vi "Drive Controller.vi"(8 "error in":errorcluster) -> ()   [LabVIEW 2019]
doc: "This VI executes continuously carrying out the current operation and responding to updates or new operation requests. It will often contain the timing or control code that is difficult to place directly in TeleOp. This VI generally opens all sensors and motors and isolates the rest of the robot code from knowing implementation details of how the operations are carried out."
uses:
  Drive Setpoints.ctl
  Drive Operations.ctl
  <vilib>/Rock Robotics/WPI/Solenoid/WPI_SolenoidChannel.ctl
  <vilib>/Rock Robotics/WPI/SafetyOutput/WPI_SafetyOutputConfigMenu.ctl
  <vilib>/Rock Robotics/WPI/ThirdParty/Phoenix-LabVIEW/Motor Controller/Controls/CTRE_Phoenix_MotorControl_ControlMode.ctl
  <vilib>/Rock Robotics/WPI/ThirdParty/Phoenix-LabVIEW/Motor Controller/Controls/CTRE_Phoenix_MotorControl_NeutralMode.ctl
  <vilib>/Rock Robotics/WPI/ThirdParty/Phoenix-LabVIEW/Motor Controller/Controls/CTRE_Phoenix_MotorControl_FeedbackDevice.ctl
  <vilib>/Rock Robotics/WPI/ThirdParty/Phoenix-LabVIEW/Motor Controller/Controls/CTRE_Phoenix_MotorControl_StatusFrameEnhanced.ctl
  <vilib>/Rock Robotics/WPI/Solenoid/WPI_SolenoidValue.ctl
  <vilib>/Rock Robotics/WPI/Solenoid/WPI_SolenoidOpenSingle.vi
  <vilib>/Rock Robotics/WPI/Solenoid/WPI_SolenoidSetEnum.vi
  <vilib>/Rock Robotics/WPI/Utilities/WPI_GetSetVariantRefNum.vi
  <vilib>/Rock Robotics/WPI/RobotDrive/WPI_RobotDriveMecanumDrive_Cartesian.vi
  <vilib>/Rock Robotics/WPI/ThirdParty/Phoenix-LabVIEW/Motor Controller/Get/CTRE_Phoenix_MotorController_GetQuadratureData.vi
panel:
  in  "output range":cluster{"output high":dbl, "output low":dbl}={"output high"=0.5, "output low"=-0.5}
  in  "PID gains":T1={"proportional gain (Kc)"=0.035, "integral time (Ti, min)"=0.0, "derivative time (Td, min)"=0.0018}
  out "Current\nCmd":string
  # ".578"
  # "Tip: It may be helpful to observe inputs and sensor values.\nYou may also want to display tuning or debugging controls."
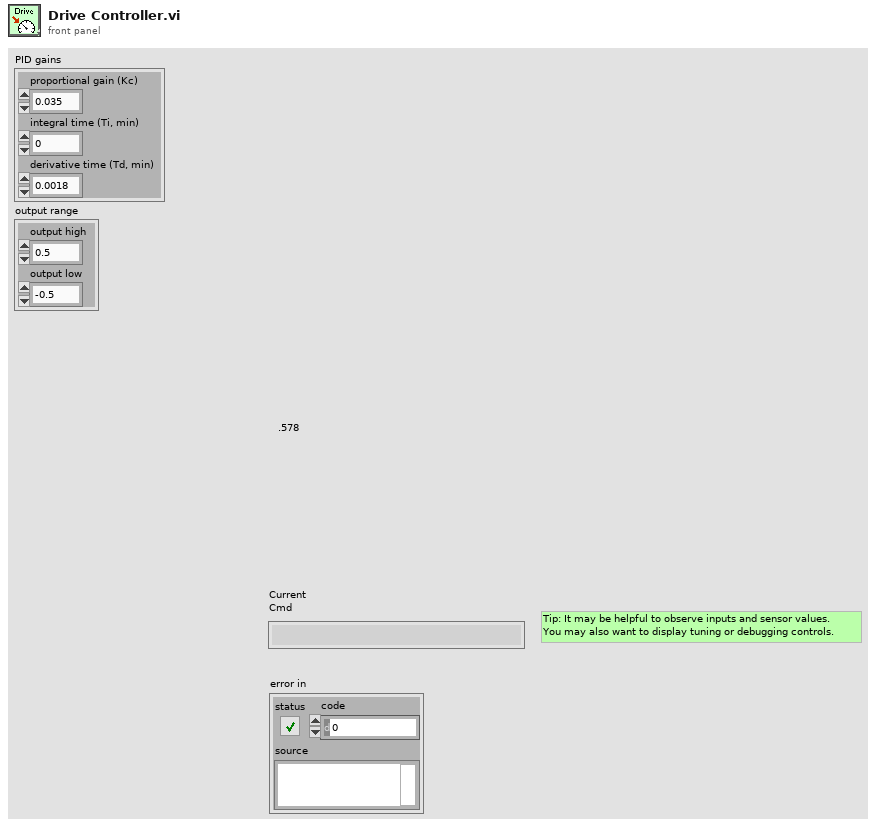
[diagram p1: front panel]
types:
  T1 = cluster{"proportional gain (Kc)":dbl, "integral time (Ti, min)":dbl, "derivative time (Td, min)":dbl}
  T2 = typedef "CTRE_Phoenix_MotorControl_StatusFrameEnhanced.ctl" = u16
  T3 = typedef "WPI_SolenoidChannel.ctl" = enum8{"Solenoid 0", "Solenoid 1", "Solenoid 2", "Solenoid 3", "Solenoid 4", "Solenoid 5", "Solenoid 6", "Solenoid 7", "Invalid"}
  T4 = typedef "CTRE_Phoenix_MotorControl_FeedbackDevice.ctl" = i8
  T5 = typedef "CTRE_Phoenix_MotorControl_NeutralMode.ctl" = enum8{"EEPROMSetting", "Override to Coast", "Override to Brake"}
  T6 = typedef "CTRE_Phoenix_MotorControl_ControlMode.ctl" = u16
  T7 = typedef "WPI_SafetyOutputConfigMenu.ctl" = enum16{"Enable", "Disable"}
  T8 = typedef "Drive Setpoints.ctl" = cluster{"Operation":T9, "X Setpoint":dbl, "Y Setpoint":dbl, "Duration":dbl, "Z Setpoint":dbl, "Tracks":bool, "Gyro":dbl, "POV":i16, "Distance(feet)":dbl, "AutoTrack Toggle":bool, "Collsision Detection":bool, "Reset Encoder":bool, "MP File Name":string}
  T9 = typedef "Drive Operations.ctl" = enum16{"Reserve", "Read Current", "Reset Motors VBus", "Motion Profile run", "Immediate Robot Centric", "Drive for Time Robot Centric", "Immediate Field Centric", "Drive For Time Field Centric", "Button Adjust", "Set Motors Motion Profile", "Reset Encoders", "Motion Profile Enable", "Drive for Distance"}
  T10 = typedef "WPI_MotorControlDeviceRef.ctl" = cluster{"DeviceStatus":errorcluster, "Type":T11, "PWM":cluster{"PWM Channel":T12, "DeadBand":T13}, "CAN":cluster{"Device Number":u8, "SetOutput VI Ref":variant, "GetOutput VI Ref":variant, "Enable VI Ref":variant, "Disable VI Ref":variant, "Data":variant}, "Invert":bool, "DIO PWM":cluster{"PWM \"Enable\" Channel":T12, "DIOChannel":T14, "PWM Rate":dbl}}
  T11 = typedef "WPI_MotorControlType.ctl" = enum16{"PWM", "CAN", "DIO PWM"}
  T12 = typedef "FPGA_DIOPWMChannel.ctl" = enum8{"PWM 0", "PWM 1", "PWM 2", "PWM 3", "PWM 4", "PWM 5", "PWM 6", "PWM 7", "PWM 8", "PWM 9", "PWM MXP 0", "PWM MXP 1", "PWM MXP 2", "PWM MXP 3", "PWM MXP 4", "PWM MXP 5", "PWM MXP 6", "PWM MXP 7", "PWM MXP 8", "PWM MXP 9", "Invalid"}
  T13 = typedef "WPI_PWMDeadband.ctl" = cluster{"Name":string, "maxPositivePwm":i32, "minPositivePwm":i32, "centerPwm":i32, "maxNegativePwm":i32, "minNegativePwm":i32, "angularRange":u16}
  T14 = typedef "FPGA_DIOChannel.ctl" = enum8{"DIO 0", "DIO 1", "DIO 2", "DIO 3", "DIO 4", "DIO 5", "DIO 6", "DIO 7", "DIO 8", "DIO 9", "DIO MXP 0", "DIO MXP 1", "DIO MXP 2", "DIO MXP 3", "DIO MXP 4", "DIO MXP 5", "DIO MXP 6", "DIO MXP 7", "DIO MXP 8", "DIO MXP 9", "DIO MXP 10", "DIO MXP 11", "DIO MXP 12", "DIO MXP 13", "DIO MXP 14", "DIO MXP 15", "SPI Port CS1", "SPI Port CS2", "SPI Port CS3", "SPI Port MISO", "SPI Port MOSI", "Invalid"}
  T15 = typedef "WPI_RobotDriveDevRef.ctl" = cluster{"DevStatus":errorcluster, "Motors[]":T10[], "Square Inputs":bool, "Max Output":dbl}
  T16 = typedef "WPI_SolenoidDevRef.ctl" = cluster{"DevStatus":errorcluster, "Pneumatics Control Module":u8, "Forward Solenoid Channel":T3, "Reverse Solenoid Channel":T3}
  T17 = typedef "Command Status Info.ctl" = cluster{"Name":string, "Status":T18, "notifier out":T19}
  T18 = typedef "Completion Status.ctl" = enum16{"Successful", "Aborted", "Incomplete"}
  T19 = typedef "Completion Notifier.ctl" = refnum<notifier>
  T20 = cluster{"SubSystem Data":T8, cluster{"Start Time (ms)":u32, "Iterations":i32}, cluster{"Command Info":T17, "Description":string, "SubSystem Data":T8, "notifier out":refnum<notifier>, "Subsystem Name":string}}
  T21 = typedef "WPI_SolenoidValue.ctl" = enum16{"Off", "On", "Forward", "Reverse"}
  T22 = cluster{"SubSystem Data":T8, cluster{"Start Time (ms)":u32, "Iterations":i32}, "Default Command Arguments":cluster{"Command Info":T17, "Description":string, "SubSystem Data":T8, "notifier out":refnum<notifier>, "Subsystem Name":string}}
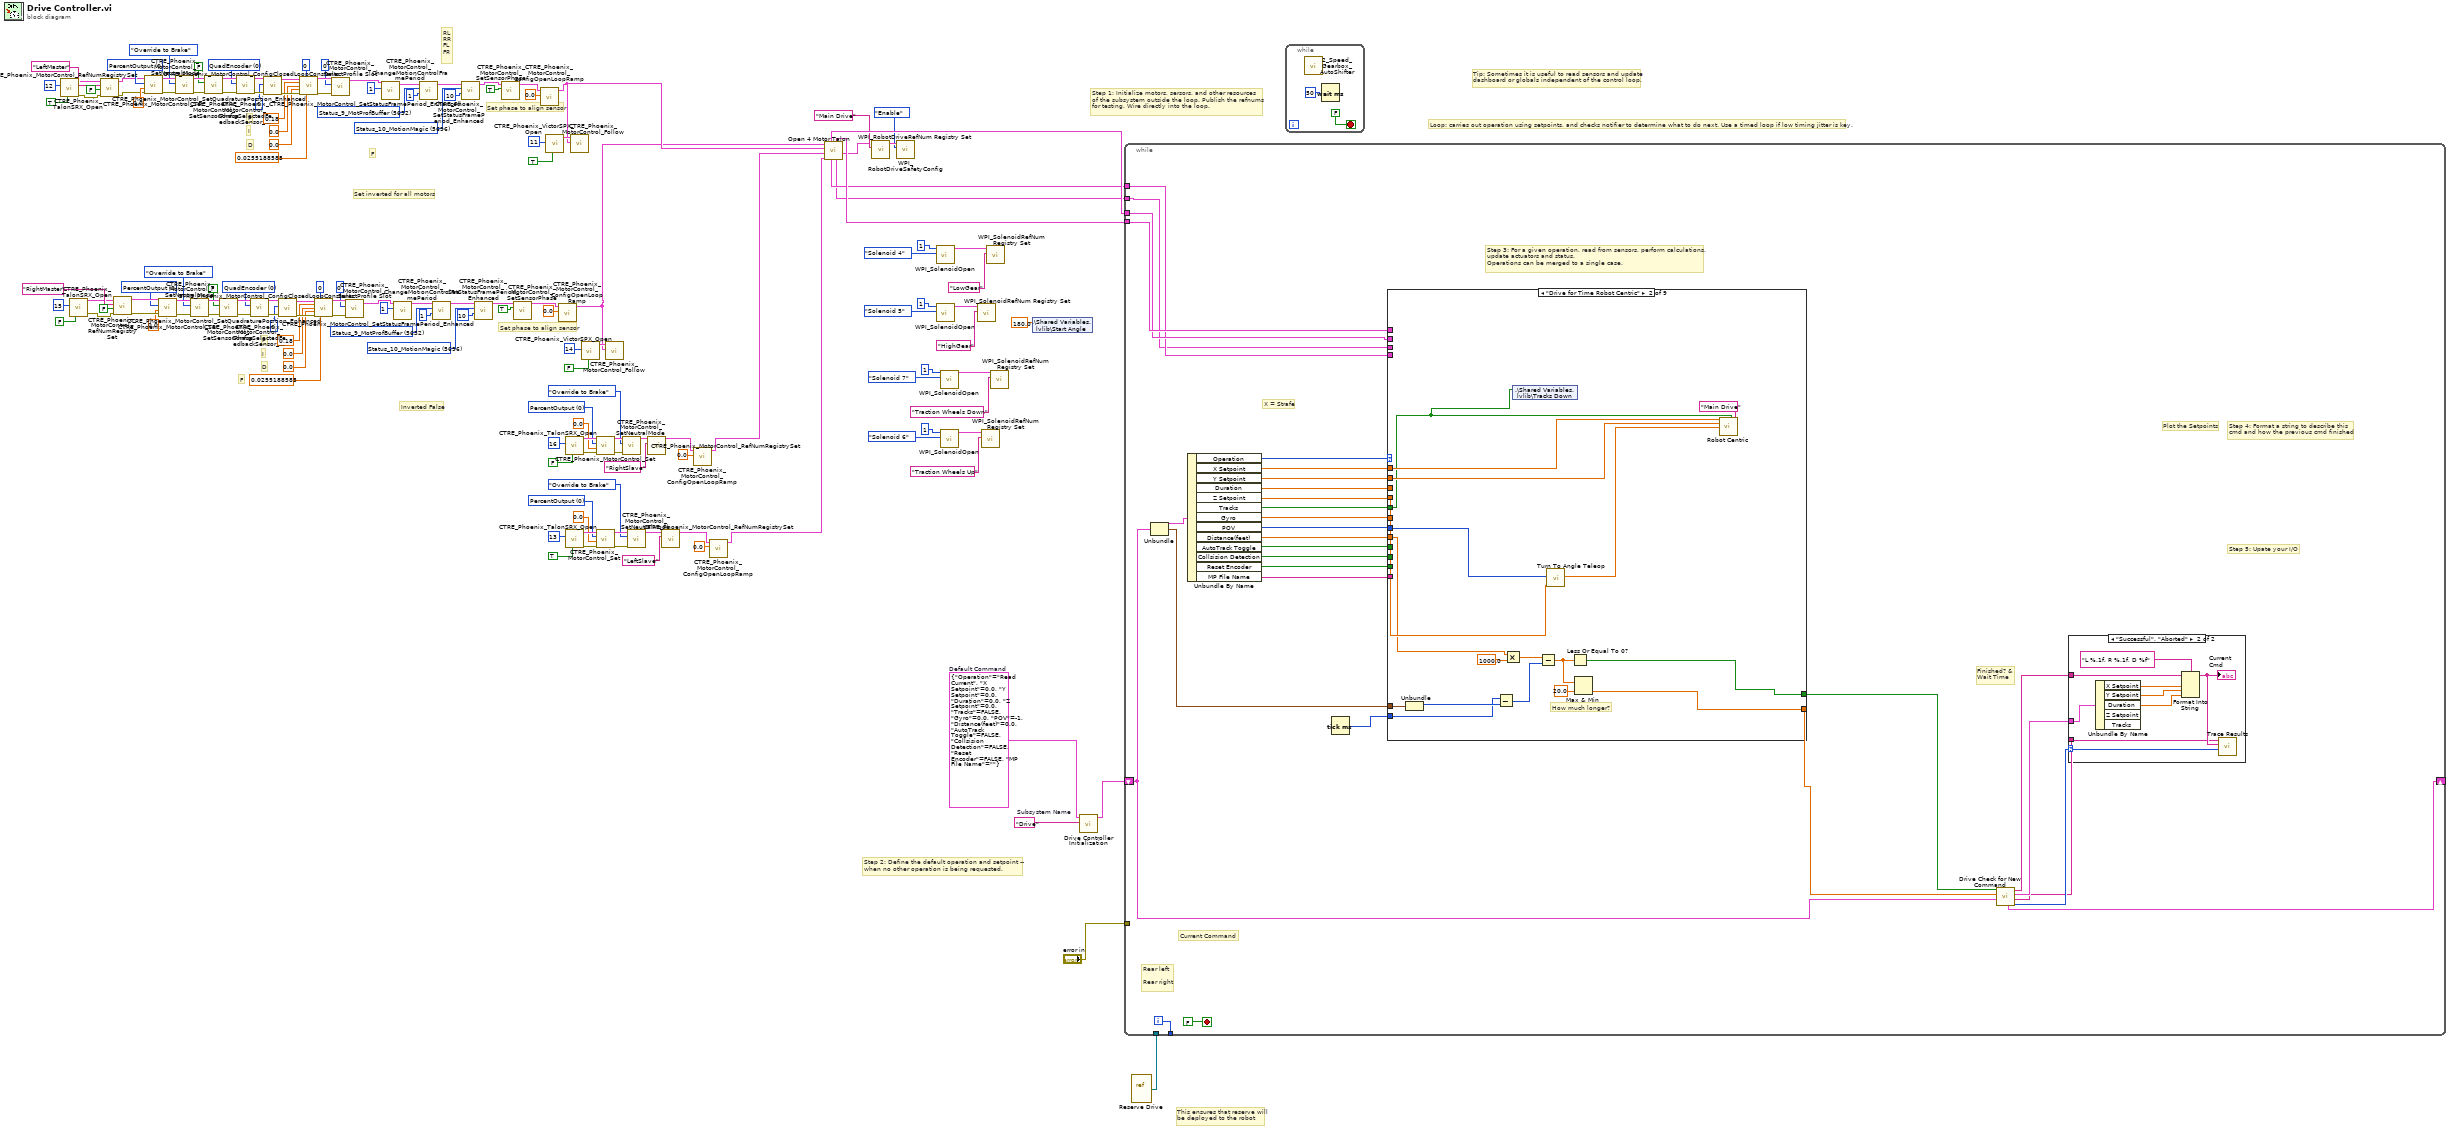
[diagram p0: block diagram]
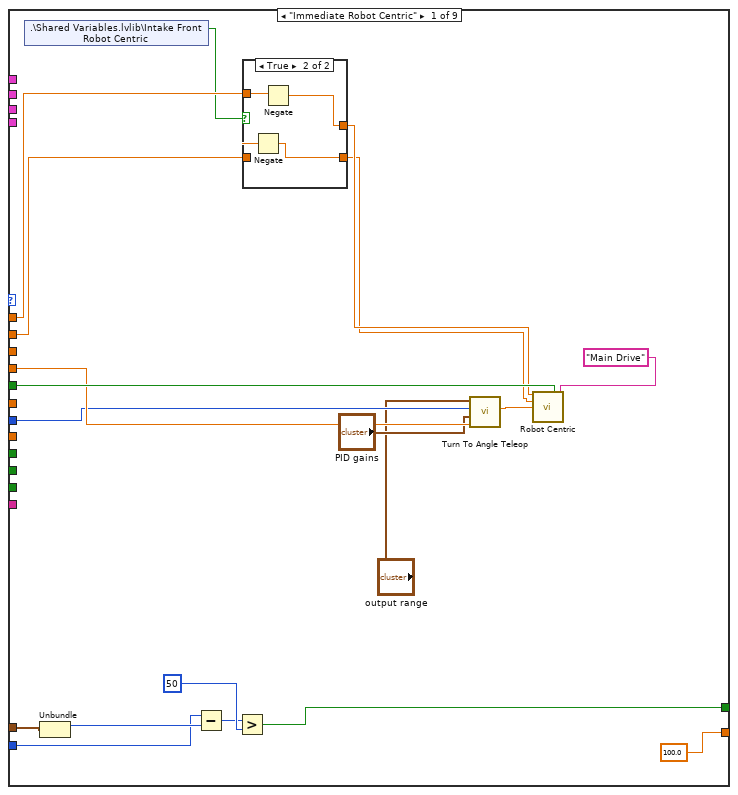
[diagram p3: hidden frame]
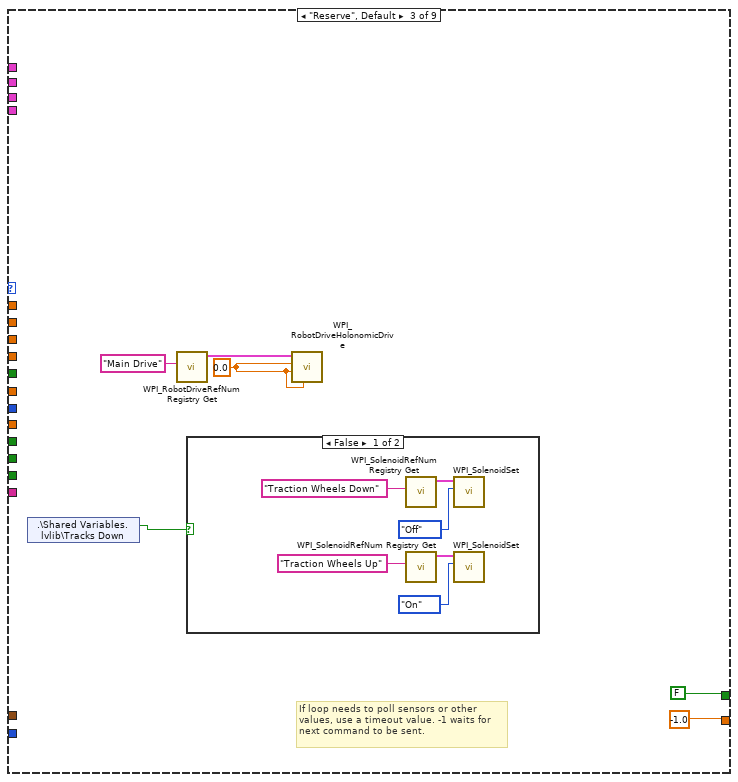
[diagram p5: hidden frame]
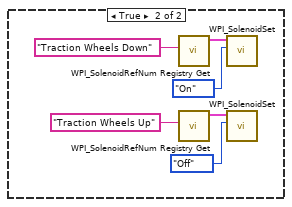
[diagram p6: hidden frame]
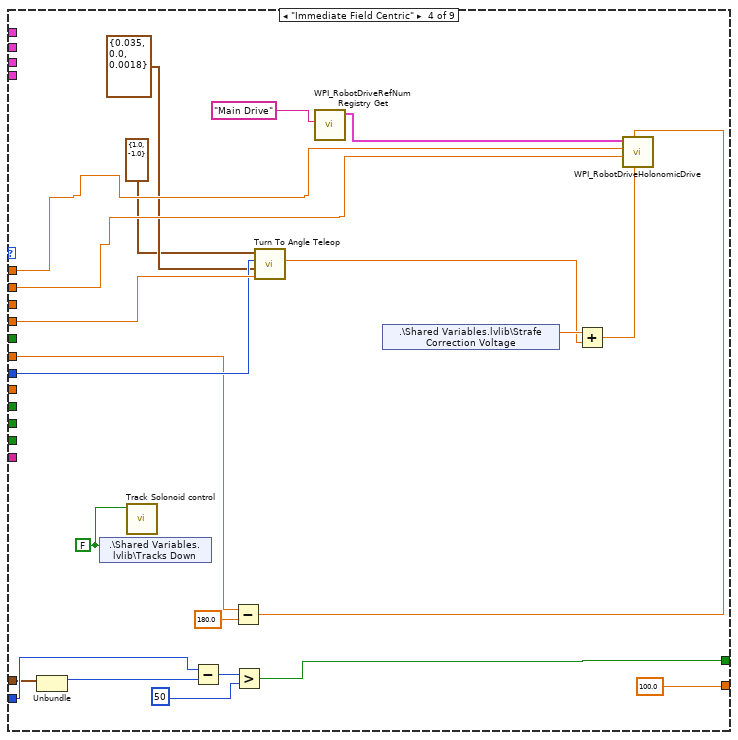
[diagram p7: hidden frame]
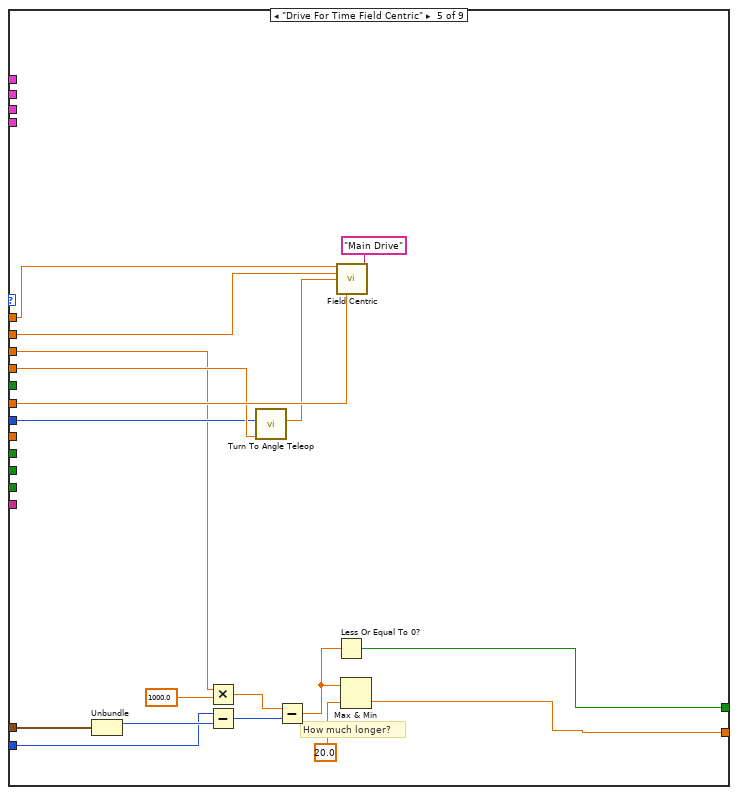
[diagram p8: hidden frame]
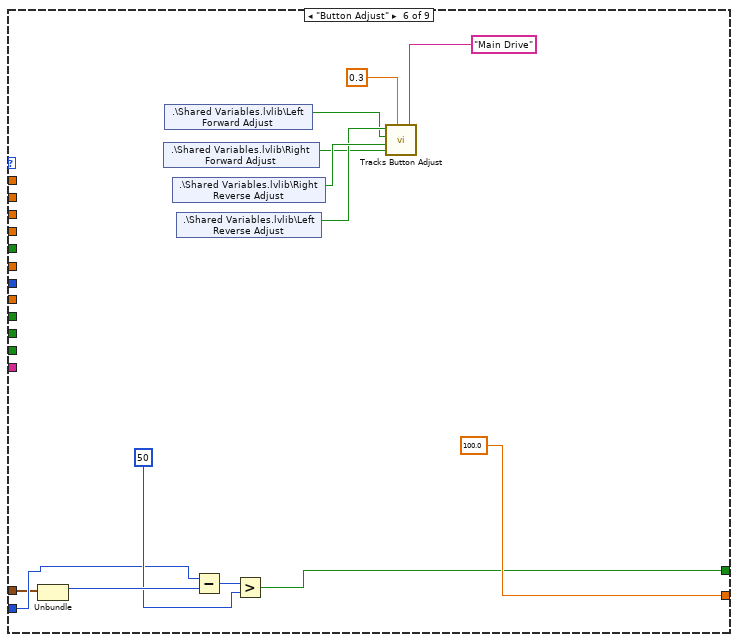
[diagram p9: hidden frame]
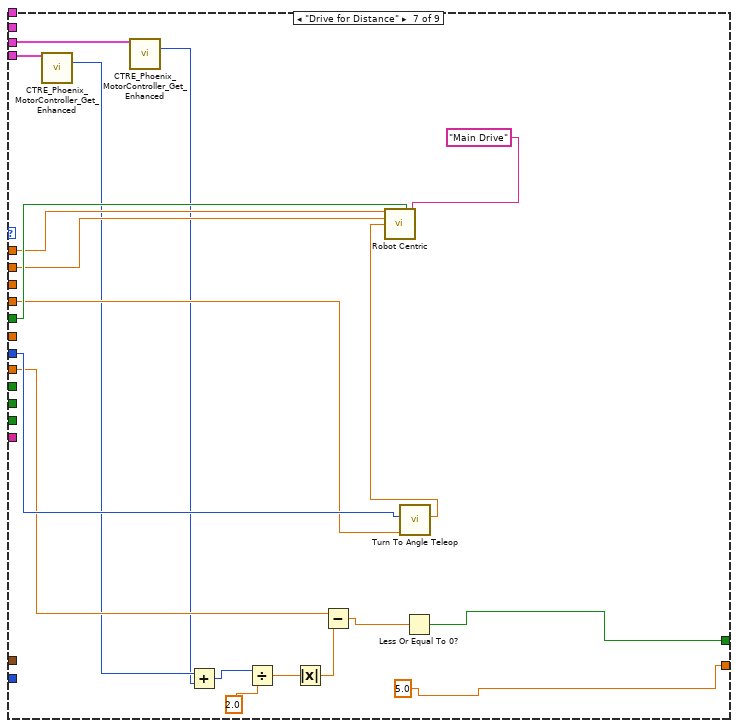
[diagram p10: hidden frame]
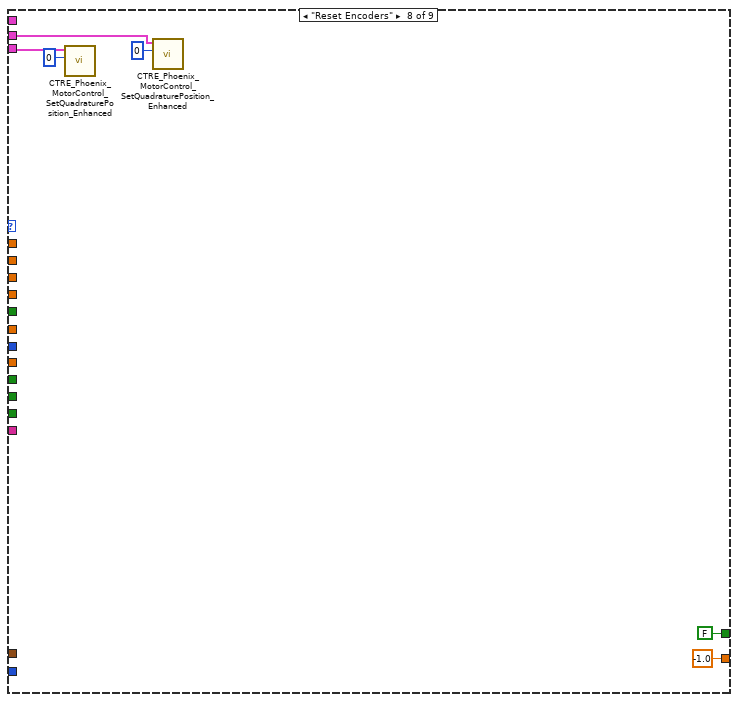
[diagram p11: hidden frame]
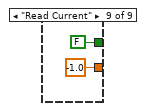
[diagram p12: hidden frame]
diagram:
  w22 = T2 5696 items=["Status_1_General"=5120, "Status_2_Feedback0"=5184, "Status_3_Quadrature"=5248, "Status_4_AinTempVbat"=5312, "Status_6_Misc"=5440, "Status_7_CommStatus"=5504, "Status_8_PulseWidth"=5568, "Status_9_MotProfBuffer"=5632, "Status_10_MotionMagic"=5696, "Status_11_UartGadgeteer"=5760, "Status_12_Feedback1"=5824, "Status_13_Base_PIDF0"=5888, "Status_14_Turn_PIDF1"=5952, "Status_15_FirmwareApiStatus"=6016] ("Status Frame")
  w24 = T2 5632 items=["Status_1_General"=5120, "Status_2_Feedback0"=5184, "Status_3_Quadrature"=5248, "Status_4_AinTempVbat"=5312, "Status_6_Misc"=5440, "Status_7_CommStatus"=5504, "Status_8_PulseWidth"=5568, "Status_9_MotProfBuffer"=5632, "Status_10_MotionMagic"=5696, "Status_11_UartGadgeteer"=5760, "Status_12_Feedback1"=5824, "Status_13_Base_PIDF0"=5888, "Status_14_Turn_PIDF1"=5952, "Status_15_FirmwareApiStatus"=6016] ("Status Frame")
  w32 = T2 5696 items=["Status_1_General"=5120, "Status_2_Feedback0"=5184, "Status_3_Quadrature"=5248, "Status_4_AinTempVbat"=5312, "Status_6_Misc"=5440, "Status_7_CommStatus"=5504, "Status_8_PulseWidth"=5568, "Status_9_MotProfBuffer"=5632, "Status_10_MotionMagic"=5696, "Status_11_UartGadgeteer"=5760, "Status_12_Feedback1"=5824, "Status_13_Base_PIDF0"=5888, "Status_14_Turn_PIDF1"=5952, "Status_15_FirmwareApiStatus"=6016] ("Status Frame")
  w34 = T2 5632 items=["Status_1_General"=5120, "Status_2_Feedback0"=5184, "Status_3_Quadrature"=5248, "Status_4_AinTempVbat"=5312, "Status_6_Misc"=5440, "Status_7_CommStatus"=5504, "Status_8_PulseWidth"=5568, "Status_9_MotProfBuffer"=5632, "Status_10_MotionMagic"=5696, "Status_11_UartGadgeteer"=5760, "Status_12_Feedback1"=5824, "Status_13_Base_PIDF0"=5888, "Status_14_Turn_PIDF1"=5952, "Status_15_FirmwareApiStatus"=6016] ("Status Frame")
  w63 = T4 0 items=["None"=-1, "QuadEncoder"=0, "Analog"=2, "Tachometer"=4, "Pulse Width Encoded Position"=8, "Sensor Sum (S0 + S1)"=9, "Sensor Difference (D0 - D1)"=10, "Remote Source 0"=11, "Remote Source 1"=12, "Software Emulated"=15] ("Feedback Device")
  w46 = T6 0 items=["PercentOutput"=0, "Position"=1, "Velocity"=2, "Current"=3, "Follower"=5, "MotionProfile"=6, "MotionMagic"=7, "MotionMagicArc"=8, "MotionProfileArc"=10, "Disabled"=15] ("Control Mode")
  w92 = T4 0 items=["None"=-1, "QuadEncoder"=0, "Analog"=2, "Tachometer"=4, "Pulse Width Encoded Position"=8, "Sensor Sum (S0 + S1)"=9, "Sensor Difference (D0 - D1)"=10, "Remote Source 0"=11, "Remote Source 1"=12, "Software Emulated"=15] ("Feedback Device")
  w77 = T6 0 items=["PercentOutput"=0, "Position"=1, "Velocity"=2, "Current"=3, "Follower"=5, "MotionProfile"=6, "MotionMagic"=7, "MotionMagicArc"=8, "MotionProfileArc"=10, "Disabled"=15] ("Control Mode")
  w108 = T6 0 items=["PercentOutput"=0, "Position"=1, "Velocity"=2, "Follower"=5, "MotionProfile"=6, "MotionMagic"=7, "MotionMagicArc"=8, "TimedPercentOutput"=9, "Disabled"=15] ("Control Mode")
  w116 = T6 0 items=["PercentOutput"=0, "Position"=1, "Velocity"=2, "Follower"=5, "MotionProfile"=6, "MotionMagic"=7, "MotionMagicArc"=8, "TimedPercentOutput"=9, "Disabled"=15] ("Control Mode")
  w153 = T8 {"Operation"=enum."Read Current", "X Setpoint"=0.0, "Y Setpoint"=0.0, "Duration"=0.0, "Z Setpoint"=0.0, "Tracks"=FALSE, "Gyro"=0.0, "POV"=-1, "Distance(feet)"=0.0, "AutoTrack Toggle"=FALSE, "Collsision Detection"=FALSE, "Reset Encoder"=FALSE, "MP File Name"=""}  # Default Command
  w154 = "Drive"  # Subsystem Name
  # "Set phase to align sensor"
  # "Set phase to align sensor"
  # "F"
  # "D"
  # "I"
  # "P"
  # "F"
  # "D"
  # "I"
  # "P"
  # "Set inverted for all motors"
  # "Inverted False"
  # "RL\nRR\nFL\nFR"
  # "This ensures that reserve will\nbe deployed to the robot"
  # "Tip: Sometimes it is useful to read sensors and update\ndashboard or globals independent of the control loop."
  # "Step 2: Define the default operation and setpoint --\nwhen no other operation is being requested."
  # "Step 1: Initialize motors, sersors, and other resources\nof the subsystem outside the loop. Publish the refnums\nfor testing. Wire directly into the loop."
  # "Loop: carries out operation using setpoints, and checks notifier to determine what to do next. Use a timed loop if low timing jitter is key."
  n1 = call <vilib>:"CTRE_Phoenix_TalonSRX_Open.vi"("Invert"=TRUE, "Device Number"=u8 12) -> ("error out"=w127:errorcluster, "CAN Talon SRX Ref"=w128:T10)  [unwired: 8 in]
  n2 = call <vilib>:"CTRE_Phoenix_TalonSRX_Open.vi"("Invert"=FALSE, "Device Number"=u8 15) -> ("error out"=w125:errorcluster, "CAN Talon SRX Ref"=w126:T10)  [unwired: 8 in]
  n3 = call <vilib>:"CTRE_Phoenix_MotorControl_RefNumRegistrySet.vi"("error in (no error)"=w127, "Test Mode Only"=FALSE, "refnum name"="LeftMaster", "PhoenixMotorControlDevRef"=w128) -> ("error out"=w75:errorcluster, "PhoenixMotorControlDevRef"=w76:T10)  [unwired: 6 in]
  n4 = call <vilib>:"CTRE_Phoenix_MotorControl_RefNumRegistrySet.vi"("error in (no error)"=w125, "Test Mode Only"=FALSE, "refnum name"="RightMaster", "PhoenixMotorControlDevRef"=w126) -> ("error out"=w48:errorcluster, "PhoenixMotorControlDevRef"=w49:T10)  [unwired: 6 in]
  n5 = call <vilib>:"CTRE_Phoenix_MotorControl_Set.vi"("error in (no error)"=w75, "Output"=0.0, "Control Mode"=w77, "PhoenixMotorControlDevRef"=w76) -> ("error out"=w96:errorcluster, "PhoenixMotorControlDevRef"=w100:T10)  [unwired: 6 in]
  n6 = call <vilib>:"CTRE_Phoenix_MotorControl_Set.vi"("error in (no error)"=w48, "Output"=0.0, "Control Mode"=w46, "PhoenixMotorControlDevRef"=w49) -> ("error out"=w67:errorcluster, "PhoenixMotorControlDevRef"=w71:T10)  [unwired: 6 in]
  n7 = call <vilib>:"CTRE_Phoenix_MotorControl_SetNeutralMode.vi"("error in (no error)"=w96, "Motor Control Neutral Mode"=CTRE_Phoenix_MotorControl_NeutralMode."Override to Brake", "PhoenixMotorControlDevRef"=w100) -> ("error out"=w98:errorcluster, "PhoenixMotorControlDevRef"=w97:T10)  [unwired: 7 in]
  n8 = call <vilib>:"CTRE_Phoenix_MotorControl_SetNeutralMode.vi"("error in (no error)"=w67, "Motor Control Neutral Mode"=CTRE_Phoenix_MotorControl_NeutralMode."Override to Brake", "PhoenixMotorControlDevRef"=w71) -> ("error out"=w69:errorcluster, "PhoenixMotorControlDevRef"=w68:T10)  [unwired: 7 in]
  n9 = call <vilib>:"CTRE_Phoenix_MotorControl_SetSensorPhase.vi"("error in (no error)"=w98, "PhaseSensor"=FALSE, "PhoenixMotorControlDevRef"=w97) -> ("error out"=w94:errorcluster, "PhoenixMotorControlDevRef"=w93:T10)  [unwired: 7 in]
  n10 = call <vilib>:"CTRE_Phoenix_MotorControl_SetSensorPhase.vi"("error in (no error)"=w69, "PhaseSensor"=FALSE, "PhoenixMotorControlDevRef"=w68) -> ("error out"=w65:errorcluster, "PhoenixMotorControlDevRef"=w64:T10)  [unwired: 7 in]
  n11 = call <vilib>:"CTRE_Phoenix_MotorControl_ConfigSelectedFeedbackSensor_Enhanced.vi"("error in (no error)"=w94, "Feedback Device"=w92, "PhoenixMotorControlDevRef"=w93) -> ("error out"=w90:errorcluster, "PhoenixMotorControlDevRef"=w91:T10)  [unwired: 7 in]
  n12 = call <vilib>:"CTRE_Phoenix_MotorControl_ConfigSelectedFeedbackSensor_Enhanced.vi"("error in (no error)"=w65, "Feedback Device"=w63, "PhoenixMotorControlDevRef"=w64) -> ("error out"=w61:errorcluster, "PhoenixMotorControlDevRef"=w62:T10)  [unwired: 7 in]
  n13 = call <vilib>:"CTRE_Phoenix_MotorControl_SetQuadraturePosition_Enhanced.vi"("error in (no error)"=w90, "New Position"=0, "PhoenixMotorControlDevRef"=w91) -> ("error out"=w87:errorcluster, "PhoenixMotorControlDevRef"=w88:T10)  [unwired: 7 in]
  n14 = call <vilib>:"CTRE_Phoenix_MotorControl_SetQuadraturePosition_Enhanced.vi"("error in (no error)"=w61, "New Position"=0, "PhoenixMotorControlDevRef"=w62) -> ("error out"=w58:errorcluster, "PhoenixMotorControlDevRef"=w59:T10)  [unwired: 7 in]
  n15 = call <vilib>:"CTRE_Phoenix_MotorControl_ConfigClosedLoopConstants.vi"("PhoenixMotorControlDevRef"=w88, "slotIdx"=0, "P"=0.18, "I"=0.0, "D"=0.0, "error in (no error)"=w87, "F"=0.0255188585) -> ("PhoenixMotorControlDevRef"=w80:T10, "error out"=w81:errorcluster)  [unwired: 7 in]
  n16 = call <vilib>:"CTRE_Phoenix_MotorControl_ConfigClosedLoopConstants.vi"("PhoenixMotorControlDevRef"=w59, "slotIdx"=0, "P"=0.18, "I"=0.0, "D"=0.0, "error in (no error)"=w58, "F"=0.0255188585) -> ("PhoenixMotorControlDevRef"=w51:T10, "error out"=w52:errorcluster)  [unwired: 7 in]
  n17 = call <vilib>:"CTRE_Phoenix_MotorControl_SelectProfile Slot.vi"("error in (no error)"=w81, "slotIdx"=0, "PhoenixMotorControlDevRef"=w80) -> ("PhoenixMotorControlDevRef"=w25:T10)  [unwired: 7 in, 1 out]
  n18 = call <vilib>:"CTRE_Phoenix_MotorControl_SelectProfile Slot.vi"("error in (no error)"=w52, "slotIdx"=0, "PhoenixMotorControlDevRef"=w51) -> ("PhoenixMotorControlDevRef"=w15:T10)  [unwired: 7 in, 1 out]
  n19 = call <vilib>:"CTRE_Phoenix_MotorControl_ChangeMotionControlFramePeriod.vi"("periodMs"=1, "PhoenixMotorControlDevRef"=w25) -> ("PhoenixMotorControlDevRef"=w29:T10)  [unwired: 8 in, 1 out]
  n20 = call <vilib>:"CTRE_Phoenix_MotorControl_ChangeMotionControlFramePeriod.vi"("periodMs"=1, "PhoenixMotorControlDevRef"=w15) -> ("PhoenixMotorControlDevRef"=w19:T10)  [unwired: 8 in, 1 out]
  n21 = call <vilib>:"CTRE_Phoenix_MotorControl_SetStatusFramePeriod_Enhanced.vi"("periodMs"=1, "Status Frame"=w34, "PhoenixMotorControlDevRef"=w29) -> ("PhoenixMotorControlDevRef"=w30:T10)  [unwired: 7 in, 1 out]
  n22 = call <vilib>:"CTRE_Phoenix_MotorControl_SetStatusFramePeriod_Enhanced.vi"("periodMs"=1, "Status Frame"=w24, "PhoenixMotorControlDevRef"=w19) -> ("PhoenixMotorControlDevRef"=w20:T10)  [unwired: 7 in, 1 out]
  n23 = call <vilib>:"CTRE_Phoenix_MotorControl_SetStatusFramePeriod_Enhanced.vi"("periodMs"=10, "Status Frame"=w32, "PhoenixMotorControlDevRef"=w30) -> ("PhoenixMotorControlDevRef"=w26:T10)  [unwired: 7 in, 1 out]
  n24 = call <vilib>:"CTRE_Phoenix_MotorControl_SetStatusFramePeriod_Enhanced.vi"("periodMs"=10, "Status Frame"=w22, "PhoenixMotorControlDevRef"=w20) -> ("PhoenixMotorControlDevRef"=w16:T10)  [unwired: 7 in, 1 out]
  n25 = call <vilib>:"CTRE_Phoenix_MotorControl_SetSensorPhase.vi"("PhaseSensor"=TRUE, "PhoenixMotorControlDevRef"=w26) -> ("PhoenixMotorControlDevRef"=w11:T10)  [unwired: 8 in, 1 out]
  n26 = call <vilib>:"CTRE_Phoenix_MotorControl_SetSensorPhase.vi"("PhaseSensor"=TRUE, "PhoenixMotorControlDevRef"=w16) -> ("PhoenixMotorControlDevRef"=w2:T10)  [unwired: 8 in, 1 out]
  n27 = call <vilib>:"CTRE_Phoenix_MotorControl_ConfigOpenLoopRamp.vi"("secondsFromNeutralToFull"=0.0, "PhoenixMotorControlDevRef"=w11) -> ("PhoenixMotorControlDevRef"=w10:T10)  [unwired: 8 in, 1 out]
  n28 = call <vilib>:"CTRE_Phoenix_VictorSPX_Open.vi"("Invert"=TRUE, "Device Number"=u8 11) -> ("CAN Talon SRX Ref"=w74:T10)  [unwired: 8 in, 1 out]
  n29 = call <vilib>:"CTRE_Phoenix_MotorControl_ConfigOpenLoopRamp.vi"("secondsFromNeutralToFull"=0.0, "PhoenixMotorControlDevRef"=w2) -> ("PhoenixMotorControlDevRef"=w1:T10)  [unwired: 8 in, 1 out]
  n30 = call <vilib>:"CTRE_Phoenix_TalonSRX_Open.vi"("Invert"=FALSE, "Device Number"=u8 16) -> ("error out"=w110:errorcluster, "CAN Talon SRX Ref"=w109:T10)  [unwired: 8 in]
  n31 = call <vilib>:"CTRE_Phoenix_TalonSRX_Open.vi"("Invert"=TRUE, "Device Number"=u8 13) -> ("error out"=w118:errorcluster, "CAN Talon SRX Ref"=w117:T10)  [unwired: 8 in]
  n32 = call <vilib>:"CTRE_Phoenix_MotorControl_Follow.vi"("Master Controller to Follow"=w10, "PhoenixMotorControlDevRef"=w74) -> ()  [unwired: 8 in, 2 out]
  n33 = call <vilib>:"CTRE_Phoenix_VictorSPX_Open.vi"("Invert"=FALSE, "Device Number"=u8 14) -> ("CAN Talon SRX Ref"=w73:T10)  [unwired: 8 in, 1 out]
  n34 = call <vilib>:"CTRE_Phoenix_MotorControl_Set.vi"("error in (no error)"=w110, "Output"=0.0, "Control Mode"=w108, "PhoenixMotorControlDevRef"=w109) -> ("error out"=w105:errorcluster, "PhoenixMotorControlDevRef"=w104:T10)  [unwired: 6 in]
  n35 = call <vilib>:"CTRE_Phoenix_MotorControl_Set.vi"("error in (no error)"=w118, "Output"=0.0, "Control Mode"=w116, "PhoenixMotorControlDevRef"=w117) -> ("error out"=w113:errorcluster, "PhoenixMotorControlDevRef"=w112:T10)  [unwired: 6 in]
  n36 = call <vilib>:"CTRE_Phoenix_MotorControl_Follow.vi"("Master Controller to Follow"=w1, "PhoenixMotorControlDevRef"=w73) -> ()  [unwired: 8 in, 2 out]
  n37 = call <vilib>:"CTRE_Phoenix_MotorControl_SetNeutralMode.vi"("error in (no error)"=w105, "Motor Control Neutral Mode"=CTRE_Phoenix_MotorControl_NeutralMode."Override to Brake", "PhoenixMotorControlDevRef"=w104) -> ("PhoenixMotorControlDevRef"=w13:T10)  [unwired: 7 in, 1 out]
  n38 = call <vilib>:"CTRE_Phoenix_MotorControl_SetNeutralMode.vi"("error in (no error)"=w113, "Motor Control Neutral Mode"=CTRE_Phoenix_MotorControl_NeutralMode."Override to Brake", "PhoenixMotorControlDevRef"=w112) -> ("PhoenixMotorControlDevRef"=w14:T10)  [unwired: 7 in, 1 out]
  n39 = call <vilib>:"CTRE_Phoenix_MotorControl_RefNumRegistrySet.vi"("refnum name"="RightSlave", "PhoenixMotorControlDevRef"=w13) -> ("PhoenixMotorControlDevRef"=w8:T10)  [unwired: 8 in, 1 out]
  n40 = call <vilib>:"CTRE_Phoenix_MotorControl_RefNumRegistrySet.vi"("refnum name"="LeftSlave", "PhoenixMotorControlDevRef"=w14) -> ("PhoenixMotorControlDevRef"=w5:T10)  [unwired: 8 in, 1 out]
  n41 = call <vilib>:"CTRE_Phoenix_MotorControl_ConfigOpenLoopRamp.vi"("secondsFromNeutralToFull"=0.0, "PhoenixMotorControlDevRef"=w8) -> ("PhoenixMotorControlDevRef"=w7:T10)  [unwired: 8 in, 1 out]
  n42 = call <vilib>:"CTRE_Phoenix_MotorControl_ConfigOpenLoopRamp.vi"("secondsFromNeutralToFull"=0.0, "PhoenixMotorControlDevRef"=w5) -> ("PhoenixMotorControlDevRef"=w4:T10)  [unwired: 8 in, 1 out]
  n43 = call "Open 4 Motor Talon.vi"("Front Right"=w4, "Front Left"=w7, "Rear Right"=w10, "Rear Left"=w1) -> ("RobotDriveDevRef"=w121:T15, "Rear Right"=w135:T10, "Front RIght"=w137:T10, "Rear Left"=w136:T10, "Front Left"=w138:T10)  [unwired: 3 in]
  n44 = call <vilib>:"WPI_RobotDriveRefNum Registry Set.vi"("refnum name"="Main Drive", "RobotDriveDevRef"=w121) -> ("RobotDriveDevRef"=w123:T15)  [unwired: 2 in, 7 out]
  n45 = call <vilib>:"WPI_RobotDriveSafetyConfig.vi"("mode"=WPI_SafetyOutputConfigMenu."Enable", "RobotDriveDevRef"=w123) -> ()  [unwired: 8 in, 2 out]
  n46 = call-poly <vilib>:"WPI_SolenoidOpen.vi"("Solenoid Channel"=WPI_SolenoidChannel."Solenoid 4", "Pneumatics Control Module (0)"=u8 1) -> ("SolenoidDevRef"=w38:T16)  [unwired: 8 in, 1 out]
  n47 = call-poly <vilib>:"WPI_SolenoidOpen.vi"("Solenoid Channel"=WPI_SolenoidChannel."Solenoid 5", "Pneumatics Control Module (0)"=u8 1) -> ("SolenoidDevRef"=w40:T16)  [unwired: 8 in, 1 out]
  n48 = call-poly <vilib>:"WPI_SolenoidOpen.vi"("Solenoid Channel"=WPI_SolenoidChannel."Solenoid 7", "Pneumatics Control Module (0)"=u8 1) -> ("SolenoidDevRef"=w143:T16)  [unwired: 8 in, 1 out]
  n49 = call-poly <vilib>:"WPI_SolenoidOpen.vi"("Solenoid Channel"=WPI_SolenoidChannel."Solenoid 6", "Pneumatics Control Module (0)"=u8 1) -> ("SolenoidDevRef"=w146:T16)  [unwired: 8 in, 1 out]
  n50 = call <vilib>:"WPI_SolenoidRefNum Registry Set.vi"("refnum name"="HighGear", "SolenoidDevRef"=w40) -> ()  [unwired: 8 in, 2 out]
  n51 = call <vilib>:"WPI_SolenoidRefNum Registry Set.vi"("refnum name"="Traction Wheels Up", "SolenoidDevRef"=w146) -> ()  [unwired: 8 in, 2 out]
  n52 = call <vilib>:"WPI_SolenoidRefNum Registry Set.vi"("refnum name"="LowGear", "SolenoidDevRef"=w38) -> ()  [unwired: 8 in, 2 out]
  n53 = call <vilib>:"WPI_SolenoidRefNum Registry Set.vi"("refnum name"="Traction Wheels Down", "SolenoidDevRef"=w143) -> ()  [unwired: 8 in, 2 out]
  n54 = shared-variable ".\\Shared Variables.lvlib\\Start Angle"(180.0 ("Start Angle")) -> ()  [unwired: 1 in, 1 out]
  n55 = call "Drive Controller Initialization.vi"("Subsystem Name"=w154, "Default Command"=w153) -> ("output cluster"=w151:T20)  [unwired: 9 in]
  n56 = vi-ref "Reserve Drive.vi"() -> (w150:refnum<vi>)
  n57 = while {
    shift-right: [w178] -> _
    shift-left: w151 -> [w167]
    tunnel: [w183] -> _
    tunnel: "error in" -> [_]
    tunnel: w150 -> [_]
    tunnel: w136 -> [w163]
    tunnel: w135 -> [w162]
    tunnel: w138 -> [w165]
    tunnel: w137 -> [w166]
    i -> [w183]
    stop <- FALSE stop-if-true
    # "X = Strafe"
    # "Rear left \n\nRear right"
    # "Step 5: Upate your I/O"
    # "Step 4: Format a string to describe this\ncmd and how the previous cmd finished"
    # "Current Command"
    # "Plot the Setpoints"
    # "Finished? &\nWait Time"
    # "Step 3: For a given operation, read from sensors, perform calculations,\nupdate actuators and status.\nOperations can be merged to a single case."
    n58 = Unbundle(w167) -> ("SubSystem Data"=w182:T8, w174:cluster{"Start Time (ms)":u32, "Iterations":i32})  [unwired: 1 out]
    n59 = Unbundle By Name(w182) -> ("Operation"=w181:T9, "X Setpoint"=w170:dbl, "Y Setpoint"=w169:dbl, "Duration"=w160:dbl, "Z Setpoint"=w173:dbl, "Tracks"=w168:bool, "Gyro"=w172:dbl, "POV"=w161:i16, "Distance(feet)"=w159:dbl, "AutoTrack Toggle"=w158:bool, "Collsision Detection"=w157:bool, "Reset Encoder"=w155:bool, "MP File Name"=w156:string)
    n60 = Tick Count (ms)() -> (millisecond timer value=w180:u32)
    n61 = case shown="\"Drive for Time Robot Centric\"" w181 {
      tunnel: [100.0 w229 -1.0 100.0 w285 100.0 5.0 ("y") -1.0 ("y") -1.0 ("y")] -> w171
      tunnel: [w207 w219 FALSE ("ignore previous (F)") w271 w284 w302 w324 FALSE ("ignore previous (F)") FALSE ("ignore previous (F)")] -> w164
      tunnel: w174 -> [w206 w234 _ w272 w287 w300 _ _ _]
      tunnel: w170 -> [w201 w226 _ w260 w282 _ w320 _ _]
      tunnel: w169 -> [w199 w225 _ w264 w294 _ w319 _ _]
      tunnel: w180 -> [w208 w232 _ w273 w286 w301 _ _ _]
      tunnel: w173 -> [w203 w222 _ w269 w279 _ w313 _ _]
      tunnel: w168 -> [w204 w224 _ _ _ _ w321 _ _]
      tunnel: w172 -> [_ _ _ w262 w281 _ _ _ _]
      tunnel: w161 -> [w197 w223 _ w268 w278 _ w315 _ _]
      tunnel: w156 -> [_ _ _ _ _ _ _ _ _]
      tunnel: w166 -> [_ _ _ _ _ _ _ _ _]
      tunnel: w165 -> [_ _ _ _ _ _ _ _ _]
      tunnel: w162 -> [_ _ _ _ _ _ w310 w331 _]
      tunnel: w163 -> [_ _ _ _ _ _ w311 w332 _]
      tunnel: w160 -> [_ _ _ _ w277 _ _ _ _]
      tunnel: w159 -> [_ w220 _ _ _ _ w312 _ _]
      tunnel: w158 -> [_ _ _ _ _ _ _ _ _]
      tunnel: w157 -> [_ _ _ _ _ _ _ _ _]
      tunnel: w155 -> [_ _ _ _ _ _ _ _ _]
      frame "Immediate Robot Centric" {
        n62 = shared-variable ".\\Shared Variables.lvlib\\Intake Front Robot Centric"() -> (w196:bool)  [unwired: 1 in, 1 out]
        n63 = Unbundle(w206) -> ("Start Time (ms)"=w209:u32)  [unwired: 1 out]
        n64 = Subtract(x=w208, y=w209) -> (x-y=w210:u32)
        n65 = Greater?(x=w210, y=u8 50 ("Left Motor")) -> (0:w207:bool)
        n66 = case shown="True" w196 {
          tunnel: w201 -> [w214 w218]
          tunnel: [w214 w217] -> w200
          tunnel: w199 -> [w213 w216]
          tunnel: [w213 w215] -> w198
          frame False {
          }
          frame True {
            n67 = Negate(x=w216) -> (-x=w215:dbl)
            n68 = Negate(x=w218) -> (-x=w217:dbl)
          }
        }
        n69 = call "Turn To Angle Teleop.vi"("Z Axis"=w203, "PID gains"="PID gains", "POV"=w197, "output range"="output range") -> ("Adjustment Voltage"=w202:dbl)  [unwired: 7 in]
        n70 = call "Robot Centric.vi"("X Axis"=w200, "Tracks Down"=w204, "Drive 1"="Main Drive", "Y Axis"=w198, "Z Axis"=w202) -> ()  [unwired: 11 in]
      }
      frame "Drive for Time Robot Centric" {
        # "How much longer?"
        n71 = Unbundle(w234) -> ("Start Time (ms)"=w233:u32)  [unwired: 1 out]
        n72 = Subtract(x=w232, y=w233) -> (x-y=w227:u32)
        n73 = Multiply(x=w220, y=1000.0) -> (x*y=w236:dbl)
        n74 = shared-variable ".\\Shared Variables.lvlib\\Tracks Down"(w224) -> ()  [unwired: 1 in, 1 out]
        n75 = Subtract(x=w236, y=w227) -> (x-y=w231:dbl)
        n76 = call "Turn To Angle Teleop.vi"("Z Axis"=w222, "POV"=w223) -> ("Adjustment Voltage"=w221:dbl)  [unwired: 9 in]
        n77 = Less Or Equal To 0?(x=w231) -> (x <= 0?=w219:bool)
        n78 = Max & Min(x=w231, y=20.0) -> (min(x,y)=w229:dbl)  [unwired: 1 out]
        n79 = call "Robot Centric.vi"("X Axis"=w226, "Tracks Down"=w224, "Drive 1"="Main Drive", "Y Axis"=w225, "Z Axis"=w221) -> ()  [unwired: 11 in]
      }
      frame "Reserve", Default {
        w238 = 0.0 ("X")
        # "If loop needs to poll sensors or other\nvalues, use a timeout value. -1 waits for\nnext command to be sent."
        n80 = shared-variable ".\\Shared Variables.lvlib\\Tracks Down"() -> (w237:bool)  [unwired: 1 in, 1 out]
        n81 = call <vilib>:"WPI_RobotDriveRefNum Registry Get.vi"("refnum name"="Main Drive" ("Drive 1")) -> ("RobotDriveDevRef"=w240:T15)  [unwired: 9 in, 1 out]
        n82 = case shown="False" w237 {
          frame False {
            n83 = call <vilib>:"WPI_SolenoidRefNum Registry Get.vi"("refnum name"="Traction Wheels Down") -> ("SolenoidDevRef"=w246:T16)  [unwired: 9 in, 1 out]
            n84 = call <vilib>:"WPI_SolenoidRefNum Registry Get.vi"("refnum name"="Traction Wheels Up") -> ("SolenoidDevRef"=w245:T16)  [unwired: 9 in, 1 out]
            n85 = call-poly <vilib>:"WPI_SolenoidSet.vi"("Value"=WPI_SolenoidValue."Off", "SolenoidDevRef"=w246) -> ()  [unwired: 8 in, 2 out]
            n86 = call-poly <vilib>:"WPI_SolenoidSet.vi"("Value"=WPI_SolenoidValue."On", "SolenoidDevRef"=w245) -> ()  [unwired: 8 in, 2 out]
          }
          frame True {
            n87 = call <vilib>:"WPI_SolenoidRefNum Registry Get.vi"("refnum name"="Traction Wheels Down") -> ("SolenoidDevRef"=w252:T16)  [unwired: 9 in, 1 out]
            n88 = call <vilib>:"WPI_SolenoidRefNum Registry Get.vi"("refnum name"="Traction Wheels Up") -> ("SolenoidDevRef"=w251:T16)  [unwired: 9 in, 1 out]
            n89 = call-poly <vilib>:"WPI_SolenoidSet.vi"("Value"=WPI_SolenoidValue."On", "SolenoidDevRef"=w252) -> ()  [unwired: 8 in, 2 out]
            n90 = call-poly <vilib>:"WPI_SolenoidSet.vi"("Value"=WPI_SolenoidValue."Off", "SolenoidDevRef"=w251) -> ()  [unwired: 8 in, 2 out]
          }
        }
        n91 = call-poly <vilib>:"WPI_RobotDriveHolonomicDrive.vi"("Rotation"=w238, "Y"=w238, "X"=w238, "RobotDriveDevRef"=w240) -> ()  [unwired: 5 in, 3 out]
      }
      frame "Immediate Field Centric" {
        w267 = FALSE ("Tracks Down")
        n92 = Unbundle(w272) -> ("Start Time (ms)"=w274:u32)  [unwired: 1 out]
        n93 = shared-variable ".\\Shared Variables.lvlib\\Tracks Down"(w267) -> ()  [unwired: 1 in, 1 out]
        n94 = call "Track Solonoid control.vi"("Manual Tracks"=w267) -> ()  [unwired: 11 in]
        n95 = Subtract(x=w273, y=w274) -> (x-y=w275:u32)
        n96 = Subtract(x=w262, y=180.0) -> (x-y=w261:dbl)
        n97 = Greater?(x=w275, y=u8 50 ("Left Motor")) -> (0:w271:bool)
        n98 = call "Turn To Angle Teleop.vi"("Z Axis"=w269, "PID gains"=T1 {"proportional gain (Kc)"=0.035, "integral time (Ti, min)"=0.0, "derivative time (Td, min)"=0.0018}, "POV"=w268, "output range"=cluster{"output high":dbl, "output low":dbl} {"output high"=1.0, "output low"=-1.0}) -> ("Adjustment Voltage"=w258:dbl)  [unwired: 7 in]
        n99 = call <vilib>:"WPI_RobotDriveRefNum Registry Get.vi"("refnum name"="Main Drive" ("Drive 1")) -> ("RobotDriveDevRef"=w265:T15)  [unwired: 9 in, 1 out]
        n100 = shared-variable ".\\Shared Variables.lvlib\\Strafe Correction Voltage"() -> (w259:dbl)  [unwired: 1 in, 1 out]
        n101 = Add(x=w259, y=w258) -> (x+y=w257:dbl)
        n102 = call-poly <vilib>:"WPI_RobotDriveHolonomicDrive.vi"("Rotation"=w257, "Gyro Angle"=w261, "Y"=w264, "X"=w260, "RobotDriveDevRef"=w265) -> ()  [unwired: 4 in, 3 out]
      }
      frame "Drive For Time Field Centric" {
        # "How much longer?"
        n103 = Unbundle(w287) -> ("Start Time (ms)"=w290:u32)  [unwired: 1 out]
        n104 = Multiply(x=w277, y=1000.0) -> (x*y=w283:dbl)
        n105 = Subtract(x=w286, y=w290) -> (x-y=w292:u32)
        n106 = call "Turn To Angle Teleop.vi"("Z Axis"=w279, "POV"=w278) -> ("Adjustment Voltage"=w280:dbl)  [unwired: 9 in]
        n107 = Subtract(x=w283, y=w292) -> (x-y=w289:dbl)
        n108 = Less Or Equal To 0?(x=w289) -> (x <= 0?=w284:bool)
        n109 = call "Field Centric.vi"("X Axis"=w282, "Drive 1"="Main Drive", "Y Axis"=w294, "Z Axis"=w280, "Gyro"=w281) -> ()  [unwired: 11 in]
        n110 = Max & Min(x=w289, y=20.0) -> (min(x,y)=w285:dbl)  [unwired: 1 out]
      }
      frame "Button Adjust" {
        n111 = Unbundle(w300) -> ("Start Time (ms)"=w306:u32)  [unwired: 1 out]
        n112 = shared-variable ".\\Shared Variables.lvlib\\Right Forward Adjust"() -> (w296:bool)  [unwired: 1 in, 1 out]
        n113 = shared-variable ".\\Shared Variables.lvlib\\Left Forward Adjust"() -> (w295:bool)  [unwired: 1 in, 1 out]
        n114 = shared-variable ".\\Shared Variables.lvlib\\Right Reverse Adjust"() -> (w298:bool)  [unwired: 1 in, 1 out]
        n115 = shared-variable ".\\Shared Variables.lvlib\\Left Reverse Adjust"() -> (w297:bool)  [unwired: 1 in, 1 out]
        n116 = Subtract(x=w301, y=w306) -> (x-y=w305:u32)
        n117 = Greater?(x=w305, y=u8 50 ("Left Motor")) -> (0:w302:bool)
        n118 = call "Tracks Button Adjust.vi"("Left Forward Adjust"=w297, "Left Reverse Adjust"=w295, "Right Forward Adjust"=w298, "Right Reverse Adjust"=w296, "Adjust Speed"=0.3, "Drive 1"="Main Drive") -> ()  [unwired: 1 in]
      }
      frame "Drive for Distance" {
        n119 = call-poly <vilib>:"CTRE_Phoenix_MotorController_Get_Enhanced.vi"("PhoenixMotorControlDevRef"=w311) -> ("Quadrature Position"=w309:i32)  [unwired: 11 in, 3 out]
        n120 = call-poly <vilib>:"CTRE_Phoenix_MotorController_Get_Enhanced.vi"("PhoenixMotorControlDevRef"=w310) -> ("Quadrature Position"=w308:i32)  [unwired: 11 in, 3 out]
        n121 = Add(x=w309, y=w308) -> (x+y=w326:i32)
        n122 = Divide(x=w326, y=2.0) -> (x/y=w323:dbl)
        n123 = Absolute Value(x=w323) -> (abs(x)=w322:dbl)
        n124 = Subtract(x=w312, y=w322) -> (x-y=w317:dbl)
        n125 = call "Turn To Angle Teleop.vi"("Z Axis"=w313, "POV"=w315) -> ("Adjustment Voltage"=w314:dbl)  [unwired: 9 in]
        n126 = call "Robot Centric.vi"("X Axis"=w320, "Tracks Down"=w321, "Drive 1"="Main Drive", "Y Axis"=w319, "Z Axis"=w314) -> ()  [unwired: 11 in]
        n127 = Less Or Equal To 0?(x=w317) -> (x <= 0?=w324:bool)
      }
      frame "Reset Encoders" {
        n128 = call <vilib>:"CTRE_Phoenix_MotorControl_SetQuadraturePosition_Enhanced.vi"("New Position"=0, "PhoenixMotorControlDevRef"=w332) -> ()  [unwired: 8 in, 2 out]
        n129 = call <vilib>:"CTRE_Phoenix_MotorControl_SetQuadraturePosition_Enhanced.vi"("New Position"=0, "PhoenixMotorControlDevRef"=w331) -> ()  [unwired: 8 in, 2 out]
      }
      frame "Read Current" {
      }
    }
    n130 = call "Drive Check for New Command.vi"("input cluster"=w167, "Wait time (ms)"=w171, "Finished?"=w164) -> ("Completion"=w179:T18, "Subsystem Name"=w175:string, "SetPoint"=w176:T8, "Initial Trace String"=w177:string, "output cluster"=w178:T22)  [unwired: 4 in]
    n131 = case shown="\"Successful\", \"Aborted\"" w179 {
      selector: w179 -> [_ w193]
      tunnel: w177 -> [_ w188]
      tunnel: w176 -> [_ w189]
      tunnel: w175 -> [_ w185]
      frame "Incomplete", Default {
        # "Continuing current command"
      }
      frame "Successful", "Aborted" {
        # "Report and setup for next command"
        n132 = Unbundle By Name(w189) -> ("X Setpoint"=w191:dbl, "Y Setpoint"=w192:dbl, "Duration"=w186:dbl)  [unwired: 2 out]
        n133 = Format Into String(format string="L %.1f, R %.1f, D %f", initial string=w188, w191, w192, w186) -> (resulting string=w187:string)  [unwired: 1 in, 1 out]
        "Current\nCmd" <- w187
        n134 = call <vilib>:"Trace Results.vi"("Status of previous command"=w193, "Description"=w187, "Subsystem"=w185) -> ()  [unwired: 9 in]
      }
    }
  }
  n135 = while {
    stop <- FALSE stop-if-true
    n136 = call "2_Speed_Gearbox_AutoShifter.vi"() -> ()  [unwired: 12 in]
    n137 = Wait (ms)(milliseconds to wait=u32 50) -> ()  [unwired: 1 out]
  }
